vi "sample2depth.vi"(0 "min":dbl, 3 "demarcate(mm)":dbl, 4 "correct(mm)":dbl, 5 "demarcate(ns)":dbl, 6 "timebase(0-4)":u32, 7 "Trigger Delay (samples)":u32, 8 "Post Trig. Samples":u32=30, 9 "Pre Trigger Samples":u32, 10 "max":dbl, 11 "sample":dbl) -> (2 "depth":dbl)   [LabVIEW 2020]
panel:
  # "pre+post trigger samples的总采样数并进行插值后的\n范围里，脉冲最大的那个位置是第几个采样点代表了深度"
  # "采样范围里最大的数"
  # "采样范围里最小的数"
  # "trigger触发后脉冲\n达到最大值的飞行时间(ns)"
  # "标定的距离(mm)"
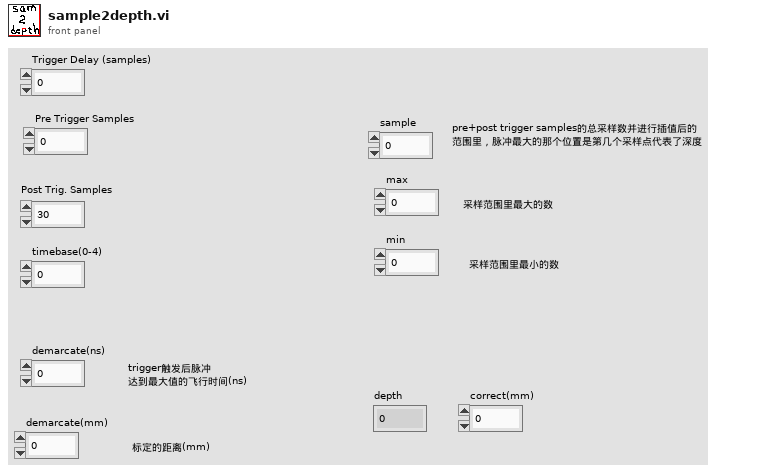
[diagram p1: front panel]
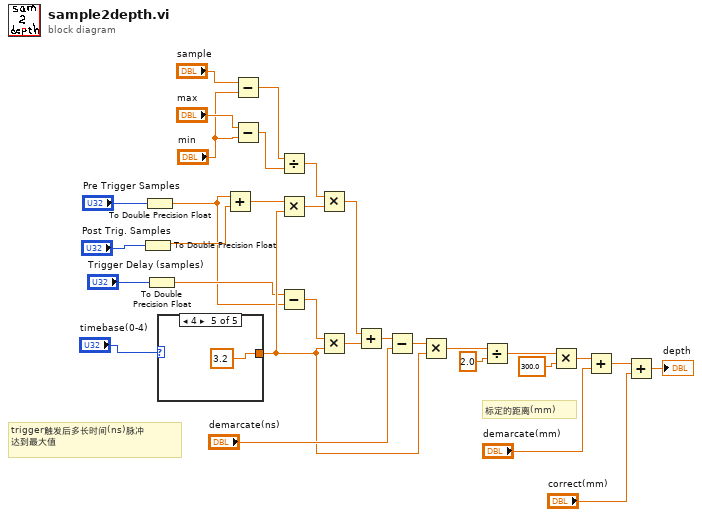
[diagram p0: block diagram]
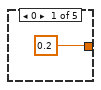
[diagram p2: hidden frame]
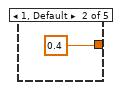
[diagram p3: hidden frame]
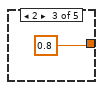
[diagram p4: hidden frame]
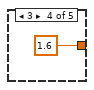
[diagram p5: hidden frame]
diagram:
  # "标定的距离(mm)"
  # "trigger触发后多长时间(ns)脉冲\n达到最大值"
  n1 = To Double Precision Float(number="Post Trig. Samples") -> (double precision float=w3:dbl)
  n2 = To Double Precision Float(number="Pre Trigger Samples") -> (double precision float=w2:dbl)
  n3 = To Double Precision Float(number="Trigger Delay (samples)") -> (double precision float=w4:dbl)
  n4 = case shown="4" "timebase(0-4)" {
    tunnel: [0.2 0.4 0.8 1.6 3.2] -> w19
    frame 0 {
    }
    frame 1, Default {
    }
    frame 2 {
    }
    frame 3 {
    }
    frame 4 {
    }
  }
  n5 = Add(x=w2, y=w3) -> (x+y=w30:dbl)
  n6 = Subtract(x="sample", y="min") -> (x-y=w8:dbl)
  n7 = Subtract(x="max", y="min") -> (x-y=w5:dbl)
  n8 = Divide(x=w8, y=w5) -> (x/y=w29:dbl)
  n9 = Multiply(x=w30, y=w19) -> (x*y=w28:dbl)
  n10 = Subtract(x=w4, y=w2) -> (x-y=w24:dbl)
  n11 = Multiply(x=w29, y=w28) -> (x*y=w27:dbl)
  n12 = Multiply(x=w24, y=w19) -> (x*y=w23:dbl)
  n13 = Add(x=w27, y=w23) -> (x+y=w21:dbl)
  n14 = Subtract(x=w21, y="demarcate(ns)") -> (x-y=w20:dbl)
  n15 = Multiply(x=w20, y=w19) -> (x*y=w18:dbl)
  n16 = Divide(x=w18, y=2.0) -> (x/y=w16:dbl)
  n17 = Multiply(x=w16, y=300.0) -> (x*y=w14:dbl)
  n18 = Add(x=w14, y="demarcate(mm)") -> (x+y=w12:dbl)
  n19 = Add(x=w12, y="correct(mm)") -> (x+y=→"depth":dbl)
